vi "Write X.vi"(8 "error in (no error)":errorcluster, 10 "X":dbl, 11 "Vec3d Class in":refnum<class "Vec3d Class.lvclass">) -> (0 "error out":errorcluster, 3 "Vec3d Class out":refnum<class "Vec3d Class.lvclass">)   [LabVIEW 2011, in "Vec3d Class.lvclass"]
uses:
  Vec3d Class.lvclass
  Vec3d Class.lvclass/Vec3d Class.ctl
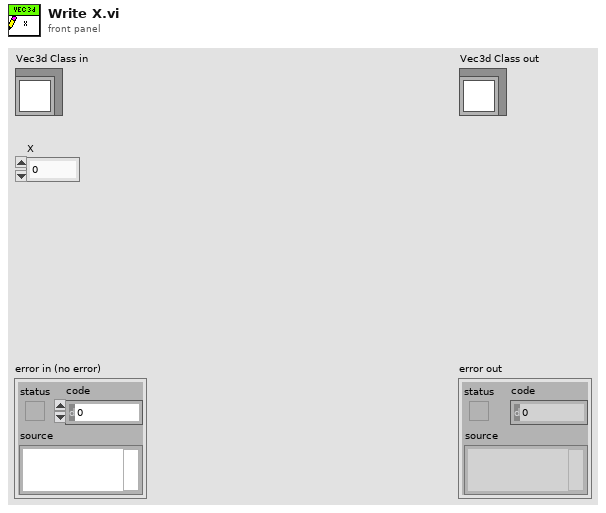
[diagram p1: front panel]
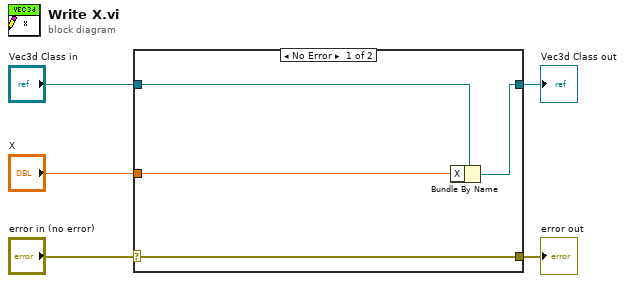
[diagram p0: block diagram]
diagram:
  n1 = case shown="No Error" "error in (no error)" {
    selector: "error in (no error)" -> [w9 w10]
    tunnel: [w9 w10] -> w4
    tunnel: [w7 w11] -> w2
    tunnel: "Vec3d Class in" -> [w8 w11]
    tunnel: "X" -> [w6 _]
    frame No Error {
      n2 = Bundle By Name(cluster=w8, "X"=w6) -> (w7:refnum<class "Vec3d Class.lvclass">)
    }
    frame Error {
    }
  }
  "error out" <- w4
  "Vec3d Class out" <- w2
